vi "程序初始化.vi"() -> (1 "数据传输队列":refnum<queue>, 2 "停止位队列":refnum<queue>, 3 "UDP网络连接输出":refnum<k16>, 4 "error out 2":errorcluster caption="错误输出", 5 "初始化数组":i32[][](array[numeric]))   [LabVIEW 2020]
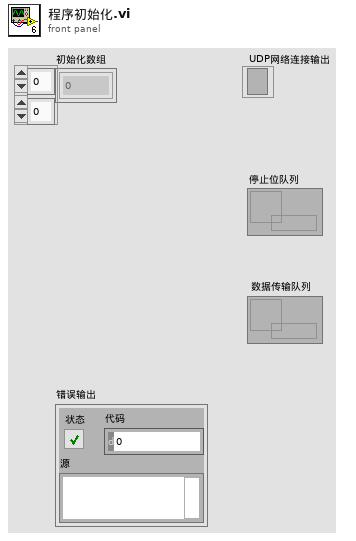
[diagram p1: front panel]
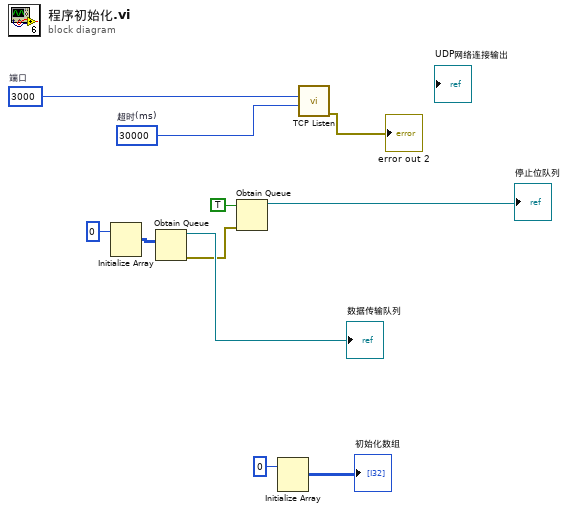
[diagram p0: block diagram]
diagram:
  w2 = 30000  # 超时(ms)
  w3 = u16 3000  # 端口
  n1 = Initialize Array(0) -> (w6:i32[][])  [unwired: 2 in]
  n2 = Obtain Queue(element data type=w6) -> (queue out=→"数据传输队列":refnum<queue>, error out=w7:errorcluster)  [unwired: 4 in, 1 out]
  n3 = Obtain Queue(element data type=TRUE, error in (no error)=w7) -> (queue out=→"停止位队列":refnum<queue>)  [unwired: 3 in, 2 out]
  n4 = Initialize Array(0) -> (→"初始化数组":i32[][])  [unwired: 2 in]
  n5 = call <vilib>:"TCP Listen.vi"("timeout ms (wait forever: -1)"=w2, "port"=w3) -> ("error out"=→"error out 2":errorcluster)  [unwired: 5 in, 4 out]
